vi "Update Progress Bar from Data Type.vi"(8 "error in":errorcluster, 11 "ESC Internal Data Structure (with types)":T1={"Test_File"=path "", "Status"="Done", "RF_Center_Freq"=0.0, "RF_Gain"=0.0, "BB_Gain"=0.0, "Error 2"="", "file_max"=0, "file_index"=0}) -> (0 "error out":errorcluster, 2 "Test Progress":dbl(slide) max=6.0 step=1.0 scale=0.0..100.0, 3 "ESC Internal Data Structure (with types) out":T1={"Test_File"=path "", "Status"="Done", "RF_Center_Freq"=0.0, "RF_Gain"=0.0, "BB_Gain"=0.0, "Error 2"="", "file_max"=0, "file_index"=0})   [LabVIEW 2017]
uses:
  TypeDef/ESC Internal Data Structure (types).ctl
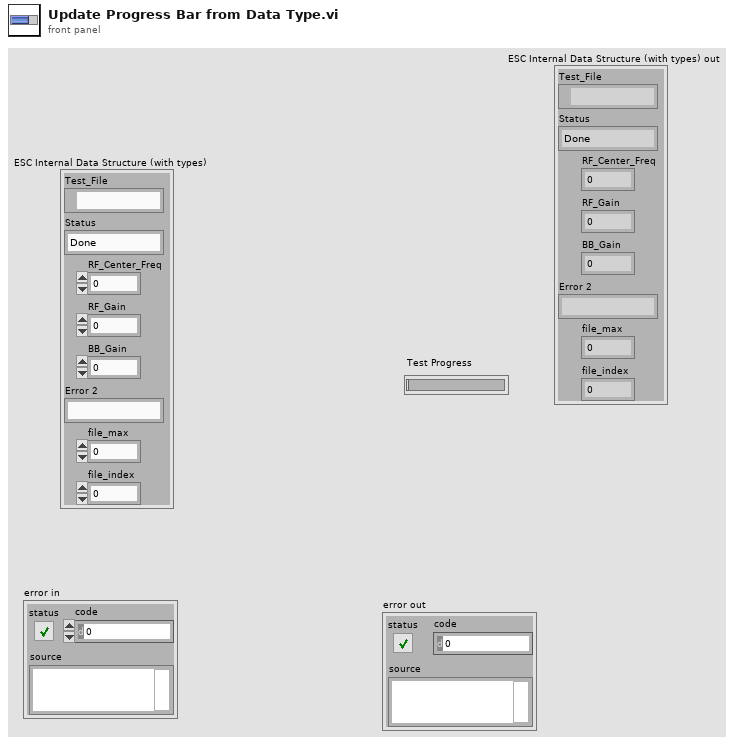
[diagram p1: front panel]
types:
  T1 = typedef "ESC Internal Data Structure (types).ctl" = cluster{"Test_File":path, "Status":string, "RF_Center_Freq":dbl, "RF_Gain":dbl, "BB_Gain":dbl, "Error 2":string, "file_max":u64, "file_index":u64}
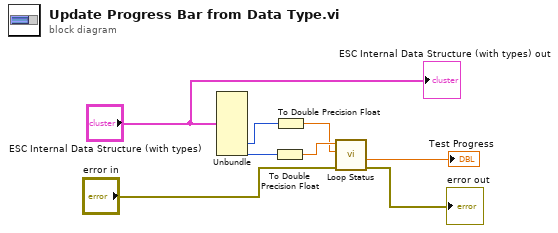
[diagram p0: block diagram]
diagram:
  n1 = Unbundle("ESC Internal Data Structure (with types)") -> ("file_max"=w8:u64, "file_index"=w7:u64)  [unwired: 6 out]
  n2 = To Double Precision Float(number=w7) -> (double precision float=w3:dbl)
  n3 = To Double Precision Float(number=w8) -> (double precision float=w2:dbl)
  n4 = call "Loop Status.vi"("error in"="error in", "total count"=w2, "current count"=w3) -> ("error out"=→"error out":errorcluster, "Percent Done"=→"Test Progress":dbl)  [unwired: 5 in, 2 out]
  "ESC Internal Data Structure (with types) out" <- "ESC Internal Data Structure (with types)"
